vi "Modbus Multi-Write STR.vi"(7 "Slave Address":u8, 8 "error in (no error)":errorcluster, 9 "Input String":string, 10 "Register Start Address":u16 format="%x", 11 "VISA resource in":refnum<visa-resource-name>) -> (0 "error out":errorcluster, 3 "VISA resource out":refnum<visa-resource-name>)   [LabVIEW 2010, in "Voegtlin_NI_SMART_Modbus_Drivers.lvlib"]
doc: "Schreibe einen beliebig langen String an die angegebene Startadresse des selektierten Geraetes. Pro Register haben zwei Zeichen platz.\nDer COM-Port muss dazu initialisiert sein (benutze\" Modbus Init.vi\")."
uses:
  Voegtlin_NI_SMART_Modbus_Drivers.lvlib
  Enums/Modbus Comm.ctl
panel:
  out "U16 input data to write\n(array)":u16[](array[numeric])
  # "Input Data"
  # "Internal Data"
  # "Output Data"
  # "(Inputmaske in HEX)"
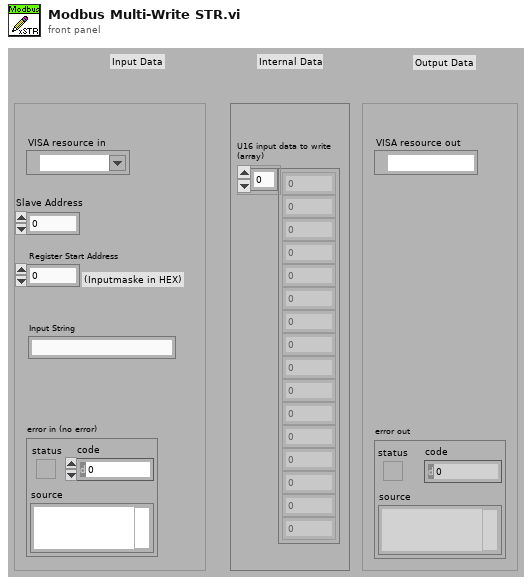
[diagram p1: front panel]
types:
  T1 = typedef "Voegtlin_NI_SMART_Modbus_Drivers.lvlib/Modbus Comm.ctl" = enum16{"Init", "Read", "Write", "Exit"}
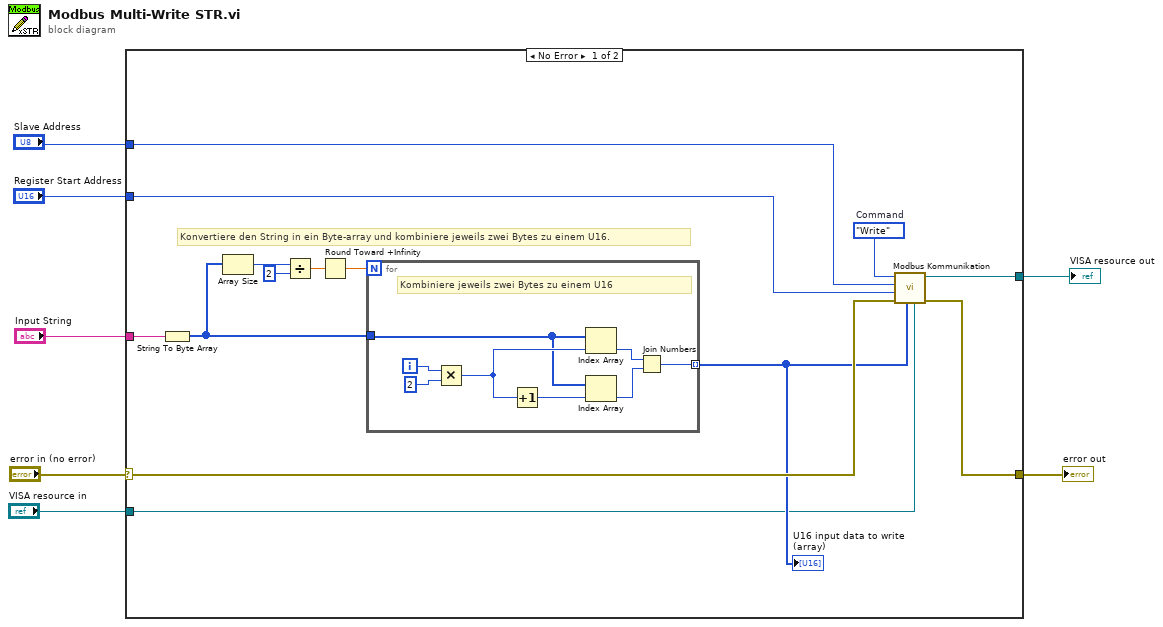
[diagram p0: block diagram]
diagram:
  n1 = case shown="No Error" "error in (no error)" {
    selector: "error in (no error)" -> [w13 w31]
    tunnel: [w20 w31] -> w7
    tunnel: "Register Start Address" -> [w11 _]
    tunnel: "Input String" -> [w19 _]
    tunnel: "Slave Address" -> [w10 _]
    tunnel: "VISA resource in" -> [w9 w30]
    tunnel: [w8 w30] -> w1
    frame No Error {
      w21 = Modbus_Comm."Write"  # Command
      # "Konvertiere den String in ein Byte-array und kombiniere jeweils zwei Bytes zu einem U16."
      n2 = String To Byte Array(string=w19) -> (unsigned byte array=w15:u8[])
      n3 = Array Size(array=w15) -> (size(s)=w16:i32)
      n4 = Divide(x=w16, y=2) -> (x/y=w17:dbl)
      n5 = Round Toward +Infinity(x=w17) -> (ceil(x): smallest int >= x=w14:dbl)
      n6 = for {
        N: w14 -> [_]
        tunnel: w15 -> [w25]
        tunnel: [w22] -> w12 mode=indexing
        i -> [w28]
        # "Kombiniere jeweils zwei Bytes zu einem U16"
        n7 = Multiply(x=w28, y=2 ("x")) -> (x*y=w27:i32)
        n8 = Increment(x=w27) -> (x+1=w26:i32)
        n9 = Index Array(array=w25, index=w27) -> (element=w24:u8)
        n10 = Index Array(array=w25, index=w26) -> (element=w23:u8)
        n11 = Join Numbers(hi=w24, lo=w23) -> ((hi.lo)=w22:u16)
      }
      "U16 input data to write\n(array)" <- w12
      n12 = call "Modbus Kommunikation.vi"("VISA resource in"=w9, "Data In / #Reads [U16]"=w12, "error in (no error)"=w13, "Register Start Address"=w11, "Slave Address"=w10, "Command"=w21) -> ("error out"=w20:errorcluster, "VISA resource out"=w8:refnum<visa-resource-name>)  [unwired: 3 in, 1 out]
    }
    frame Error {
    }
  }
  "error out" <- w7
  "VISA resource out" <- w1
